vi "Set VSingle Mode.vi"(10 "OSC1 IP:":refnum<visa-resource-name>="DSOS404", 11 "Acquistion Mode":u16(ring)=1 items=["Run/Stop", "Single"]) -> ()   [LabVIEW 2018]
uses:
  <instrlib>/Agilent 90000 Series/Agilent 90000 Series.lvlib
panel:
  out "error out":errorcluster
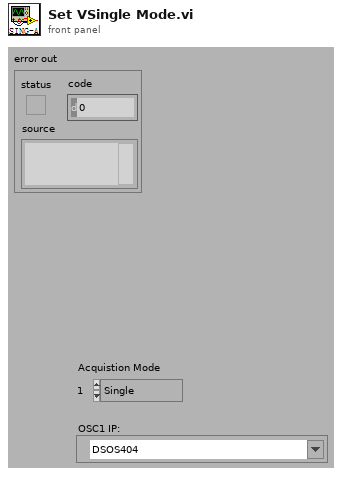
[diagram p1: front panel]
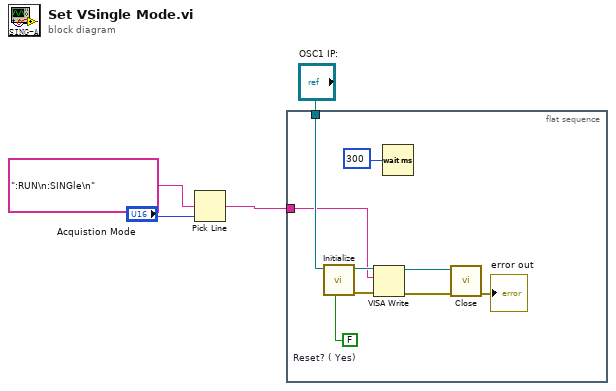
[diagram p0: block diagram]
diagram:
  n1 = Pick Line(multi-line string=":RUN\n:SINGle\n", line index="Acquistion Mode") -> (output string=w1:string)  [unwired: 1 in]
  n2 = flat-sequence {
    tunnel: w1 -> [w8]
    tunnel: "OSC1 IP:" -> [w12]
    frame #0 {
      w13 = FALSE  # Reset? ( Yes)
      n3 = call <instrlib>:"Initialize.vi"("Reset (True)"=w13, "VISA resource name"=w12) -> ("error out"=w7:errorcluster, "VISA resource name out"=w11:refnum<visa-resource-name>)  [unwired: 8 in]
      n4 = VISA Write(VISA resource name=w11, write buffer=w8, error in (no error)=w7) -> (VISA resource name out=w10:refnum<visa-resource-name>, error out=w6:errorcluster)  [unwired: 1 out]
      n5 = Wait (ms)(milliseconds to wait=u32 300) -> ()  [unwired: 1 out]
      n6 = call <instrlib>:"Close.vi"("error in (no error)"=w6, "VISA resource name"=w10) -> ("error out"=→"error out":errorcluster)  [unwired: 9 in]
    }
  }
